vi "Ih_Image_Tiling.vi"(8 "error in (no error)":errorcluster, 10 "2D array in (LCOS size buf)":u8[][](array[numeric]), 11 "2D array in":u8[][](array[numeric])) -> (0 "error out":errorcluster, 3 "2D array out":u8[][](array[numeric]))   [LabVIEW 2017]
uses:
  SLM_Control_VI_source/Image_Control.dll
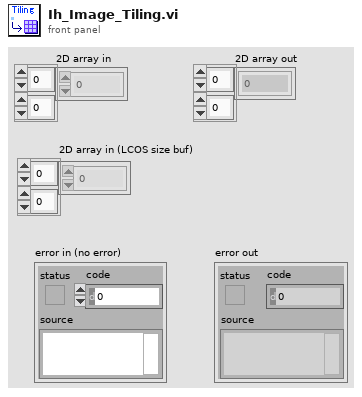
[diagram p1: front panel]
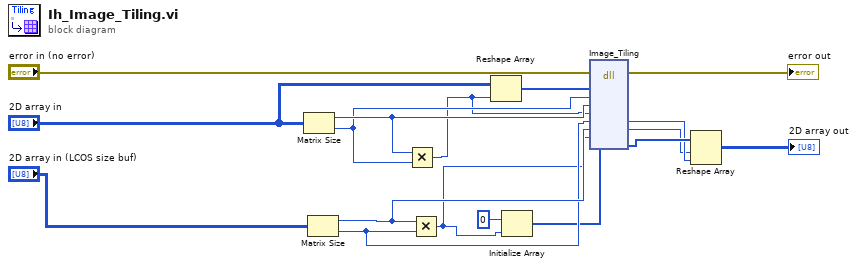
[diagram p0: block diagram]
diagram:
  n1 = Matrix Size(0:"2D array in") -> (1:w14:i32, 2:w11:i32)
  n2 = Matrix Size(0:"2D array in (LCOS size buf)") -> (1:w9:i32, 2:w8:i32)
  n3 = Multiply(x=w14, y=w11) -> (x*y=w7:i32)
  n4 = Multiply(x=w9, y=w8) -> (x*y=w6:i32)
  n5 = Reshape Array("2D array in", w7) -> (w12:u8[])
  n6 = Initialize Array(u8 0 ("要素"), w6) -> (w5:u8[])
  n7 = dll-call lib="C:/Users/hs5921/Desktop/SLM_Control_VI_source/Image_Control.dll" fn="Image_Tiling"(error in="error in (no error)", "1DArrayIn"=w12, "X_pixel_in"=w11, "Y_pixel_in"=w14, "inputDataSize"=w7, "X_pixel_target"=w8, "Y_pixel_target"=w9, "targetDataSize"=w6, "1DArrayOut"=w5) -> (error out=→"error out":errorcluster, "X_pixel_target"=w3:i32, "Y_pixel_target"=w2:i32, "1DArrayOut"=w4:u8[])  [unwired: 8 in, 1 out]
  n8 = Reshape Array(w4, w2, w3) -> (→"2D array out":u8[][])
